vi "WordStr2WordValue.vi"(8 "error in (no error)":errorcluster, 11 "Word":string) -> (0 "error out":errorcluster, 3 "Word Value":i32)   [LabVIEW 2016, in "Motor Base.lvlib" / "Motor Base.lvclass"]
uses:
  Motor Base.lvclass
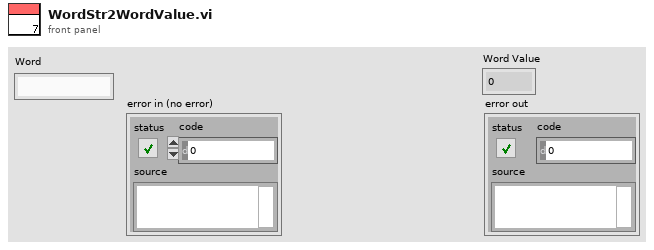
[diagram p1: front panel]
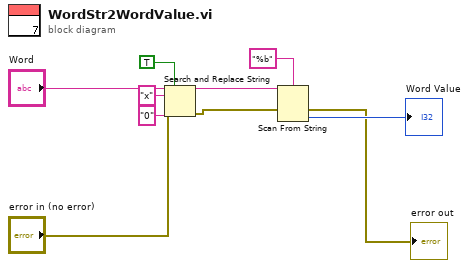
[diagram p0: block diagram]
diagram:
  n1 = Search and Replace String(replace all?=TRUE ("replace all? (F)"), input string="Word", search string="x", replace string="0" ("replace string (\"\")"), error in="error in (no error)") -> (result string=w5:string, error out=w2:errorcluster)  [unwired: 3 in, 2 out]
  n2 = Scan From String(format string="%b", input string=w5, error in=w2) -> (error out=→"error out":errorcluster, output 1=→"Word Value":i32)  [unwired: 2 in, 2 out]
